vi "Terminal-Core-InitializeQueues.vi"(1 "comand (Initialize)":enum16{"UnInitialize", "Initialize"}(ring), 5 "error in (no error)":errorcluster caption="错误输入（无错误）") -> (13 "error out":errorcluster caption="错误输出", 14 "CmdQRef":refnum<queue>, 15 "ModbusMsgQRef":refnum<queue>, 16 "GuiModbusQRef":refnum<queue>, 17 "DataQRef":refnum<queue>, 18 "UdpQRef":refnum<queue>, 19 "ErrorQRef":refnum<queue>)   [LabVIEW 2014]
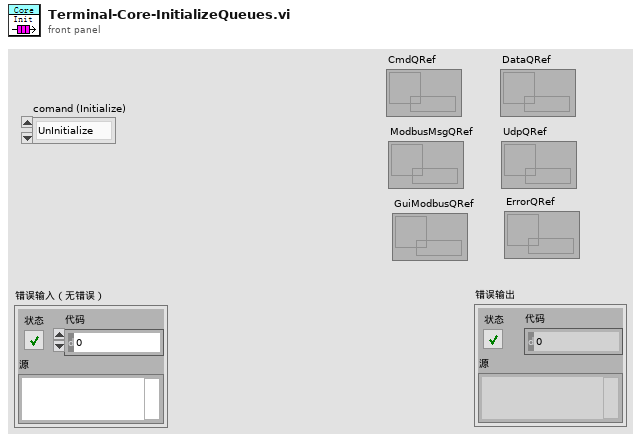
[diagram p1: front panel]
types:
  T1 = cluster{"设备名":string, "时间":timestamp, "数据":sgl[][], "通道长度":i32[], "次数":i32}
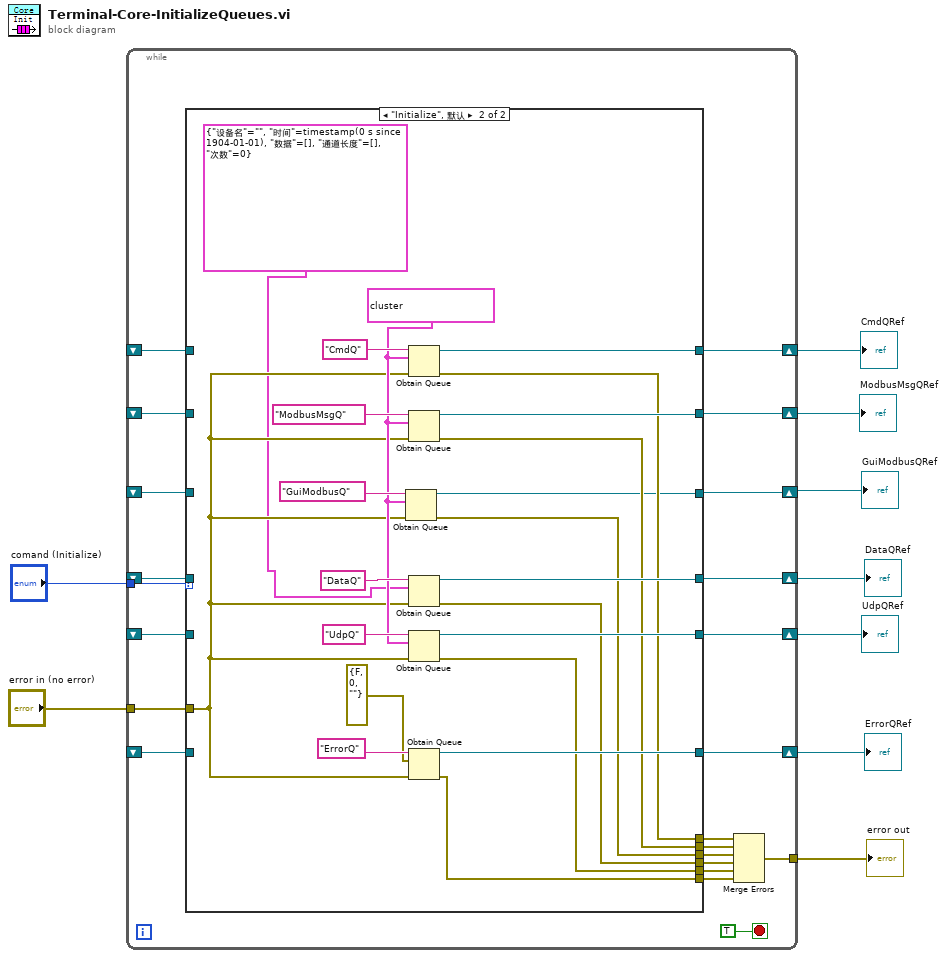
[diagram p0: block diagram]
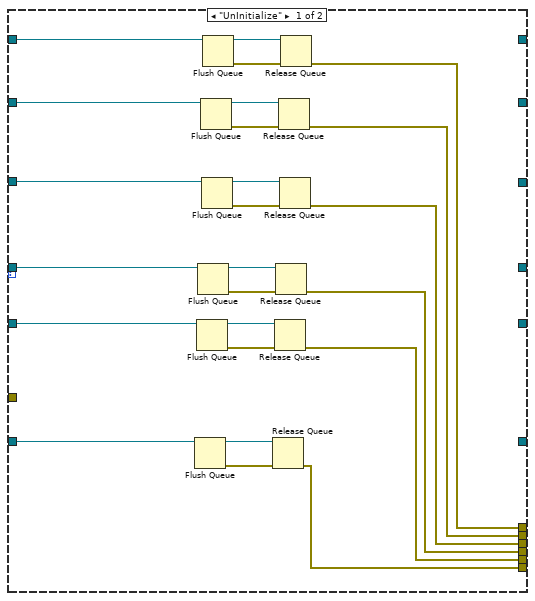
[diagram p2: hidden frame]
diagram:
  n1 = while {
    shift-right: [w30] -> w5
    shift-left: _ -> [w29]
    tunnel: "comand (Initialize)" -> [w28]
    tunnel: "error in (no error)" -> [w27]
    shift-right: [w24] -> w4
    shift-left: _ -> [w18]
    shift-right: [w25] -> w1
    shift-left: _ -> [w17]
    shift-right: [w26] -> w3
    shift-left: _ -> [w16]
    shift-right: [w23] -> w6
    shift-left: _ -> [w15]
    tunnel: [w19] -> w7
    shift-right: [w14] -> w2
    shift-left: _ -> [w13]
    stop <- TRUE stop-if-true
    n2 = case shown="\"Initialize\", 默认" w28 {
      tunnel: [_ w63] -> w30
      tunnel: w29 -> [w45 _]
      tunnel: w27 -> [_ w58]
      tunnel: [_ w71] -> w26
      tunnel: [_ w70] -> w25
      tunnel: [_ w69] -> w24
      tunnel: [_ w68] -> w23
      tunnel: [w36 w62] -> w22
      tunnel: [w37 w67] -> w12
      tunnel: [w38 w65] -> w21
      tunnel: [w39 w64] -> w20
      tunnel: [w40 w66] -> w11
      tunnel: w18 -> [w44 _]
      tunnel: w17 -> [w43 _]
      tunnel: w16 -> [w42 _]
      tunnel: w15 -> [w41 _]
      tunnel: [_ w61] -> w14
      tunnel: w13 -> [w33 _]
      tunnel: [w32 w57] -> w10
      frame "UnInitialize" {
        n3 = Flush Queue(queue=w41) -> (queue out=w47:refnum<queue>, error out=w46:errorcluster)  [unwired: 1 in, 1 out]
        n4 = Flush Queue(queue=w42) -> (queue out=w49:refnum<queue>, error out=w48:errorcluster)  [unwired: 1 in, 1 out]
        n5 = Flush Queue(queue=w43) -> (queue out=w51:refnum<queue>, error out=w50:errorcluster)  [unwired: 1 in, 1 out]
        n6 = Flush Queue(queue=w44) -> (queue out=w53:refnum<queue>, error out=w52:errorcluster)  [unwired: 1 in, 1 out]
        n7 = Flush Queue(queue=w33) -> (queue out=w35:refnum<queue>, error out=w34:errorcluster)  [unwired: 1 in, 1 out]
        n8 = Flush Queue(queue=w45) -> (queue out=w55:refnum<queue>, error out=w54:errorcluster)  [unwired: 1 in, 1 out]
        n9 = Release Queue(queue=w47, error in (no error)=w46) -> (error out=w40:errorcluster)  [unwired: 1 in, 2 out]
        n10 = Release Queue(queue=w49, error in (no error)=w48) -> (error out=w39:errorcluster)  [unwired: 1 in, 2 out]
        n11 = Release Queue(queue=w51, error in (no error)=w50) -> (error out=w38:errorcluster)  [unwired: 1 in, 2 out]
        n12 = Release Queue(queue=w53, error in (no error)=w52) -> (error out=w37:errorcluster)  [unwired: 1 in, 2 out]
        n13 = Release Queue(queue=w35, error in (no error)=w34) -> (error out=w32:errorcluster)  [unwired: 1 in, 2 out]
        n14 = Release Queue(queue=w55, error in (no error)=w54) -> (error out=w36:errorcluster)  [unwired: 1 in, 2 out]
      }
      frame "Initialize", Default {
        w59 = cluster{variant, string} {variant, "Cmd::Initialize"}
        n15 = Obtain Queue(name (unnamed)="GuiModbusQ" ("名称（未命名）"), element data type=w59, error in (no error)=w58) -> (queue out=w61:refnum<queue>, error out=w57:errorcluster)  [unwired: 2 in, 1 out]
        n16 = Obtain Queue(name (unnamed)="CmdQ" ("名称（未命名）"), element data type=w59, error in (no error)=w58) -> (queue out=w63:refnum<queue>, error out=w62:errorcluster)  [unwired: 2 in, 1 out]
        n17 = Obtain Queue(name (unnamed)="ModbusMsgQ" ("名称（未命名）"), element data type=w59, error in (no error)=w58) -> (queue out=w69:refnum<queue>, error out=w67:errorcluster)  [unwired: 2 in, 1 out]
        n18 = Obtain Queue(name (unnamed)="DataQ" ("名称（未命名）"), element data type=T1 {"设备名"="", "时间"=timestamp(0 s since 1904-01-01), "数据"=[], "通道长度"=[], "次数"=0}, error in (no error)=w58) -> (queue out=w70:refnum<queue>, error out=w65:errorcluster)  [unwired: 2 in, 1 out]
        n19 = Obtain Queue(name (unnamed)="UdpQ" ("名称（未命名）"), element data type=w59, error in (no error)=w58) -> (queue out=w71:refnum<queue>, error out=w64:errorcluster)  [unwired: 2 in, 1 out]
        n20 = Obtain Queue(name (unnamed)="ErrorQ" ("名称（未命名）"), element data type=errorcluster {"status"=FALSE, "code"=0, "source"=""} ("错误常量"), error in (no error)=w58) -> (queue out=w68:refnum<queue>, error out=w66:errorcluster)  [unwired: 2 in, 1 out]
      }
    }
    n21 = Merge Errors(w22, w12, w10, w21, w20, w11) -> (w19:errorcluster)
  }
  "error out" <- w7
  "ErrorQRef" <- w6
  "CmdQRef" <- w5
  "ModbusMsgQRef" <- w4
  "UdpQRef" <- w3
  "GuiModbusQRef" <- w2
  "DataQRef" <- w1
